vi "get-histogram.vi"() -> (0 "IntegralCount":u32, 1 "Histogram":u32[](array[numeric]))   [LabVIEW 2015]
uses:
  phlib.dll
panel:
  out "Overflow":bool
  out "Flags":i32 format="%.0b"
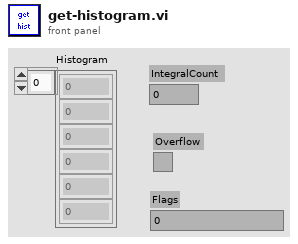
[diagram p1: front panel]
types:
  T1 = cluster{"initialized":bool, "devidx":i32, "Ch0 Level":i32, "Ch0 ZeroX":i32, "Ch1 Level":i32, "Ch1 ZeroX":i32, "sync rate":i32, "resolution":i32, "acq time":i32, "acq rate":i32, "# bins":u32, "Bin size":enum16{"1", "2", "4", "8", "16", "32", "64", "128"}, "min photons":u32, "truncate":u32}
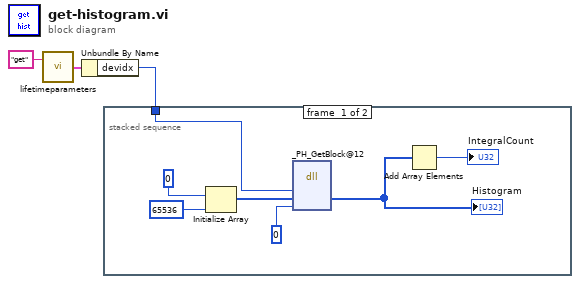
[diagram p0: block diagram]
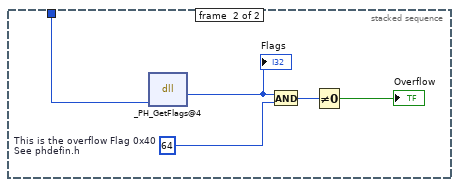
[diagram p2: hidden frame]
diagram:
  n1 = call "lifetimeparameters.vi"("command"="get") -> ("Params out"=w2:T1)  [unwired: 1 in]
  n2 = Unbundle By Name(w2) -> ("devidx"=w1:i32)
  n3 = stacked-sequence {
    tunnel: w1 -> [w5 w11]
    frame #0 {
      n4 = Initialize Array "Initialize Array"(u32 0, 65536) -> (w7:u32[])
      n5 = dll-call lib="phlib.dll" fn="_PH_GetBlock@12" label="PH_GetBlock"("devidx"=w5, "Chcount"=w7, "block"=0) -> ("Chcount"=w4:u32[])  [unwired: 6 in, 2 out]
      "Histogram" <- w4
      n6 = Add Array Elements(numeric array=w4) -> (sum=→"IntegralCount":u32)
    }
    frame #1 {
      w15 = 64  # This is the overflow Flag 0x40 See phdefin.h
      n7 = dll-call lib="phlib.dll" fn="_PH_GetFlags@4" label="PH_GetFlags"("devidx"=w11) -> (w14:i32)  [unwired: 4 in, 2 out]
      "Flags" <- w14
      n8 = And(x=w14, y=w15) -> (x .and. y?=w12:i32)
      n9 = Not Equal To 0?(x=w12) -> (x != 0?=→"Overflow":bool)
    }
  }
